vi "FGV_UserMenu.vi"(7 "Command":enum16{"Initialize", "Set", "Get"}(ring), 10 "Use Info":string, 11 "VI Refnum":refnum<vi>) -> (2 "String":string)   [LabVIEW 2017]
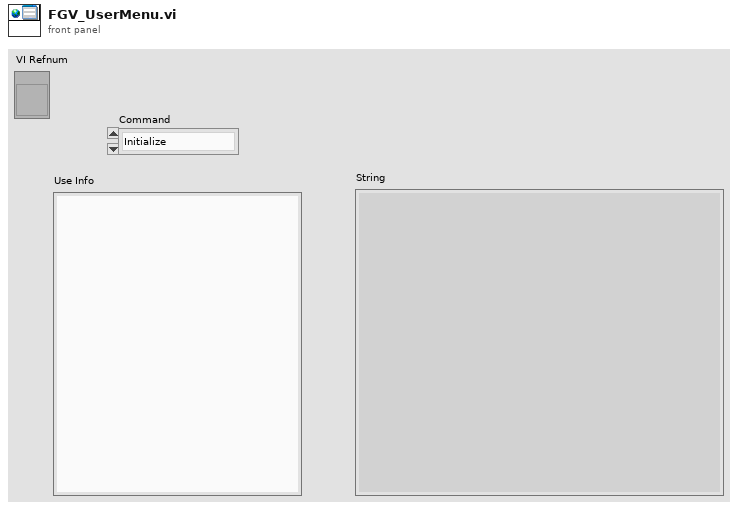
[diagram p1: front panel]
types:
  T1 = cluster{"VI Refnum":refnum<vi>, "Use Info":string}[]
  T2 = cluster{"VI Refnum":refnum<vi>, "Use Info":string}
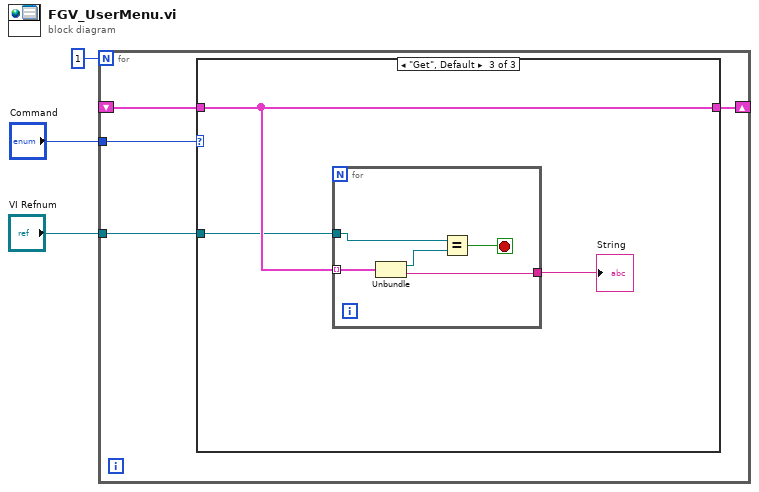
[diagram p0: block diagram]
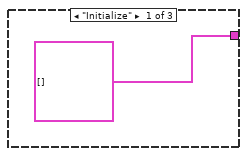
[diagram p2: hidden frame]
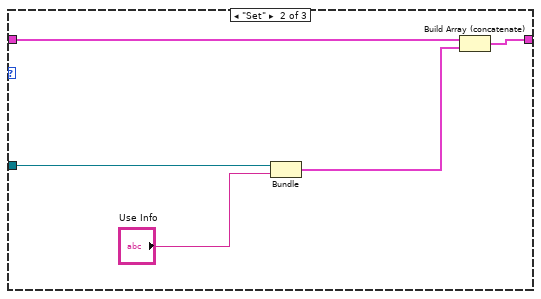
[diagram p3: hidden frame]
diagram:
  n1 = for {
    N: 1 -> [_]
    shift-right: [w4] -> _
    shift-left: _ -> [w7]
    tunnel: "Command" -> [w6]
    tunnel: "VI Refnum" -> [w5]
    n2 = case shown="\"Get\", Default" w6 {
      tunnel: w7 -> [_ w9 w16]
      tunnel: w5 -> [_ w13 w15]
      tunnel: [T1 [] w10 w16] -> w4
      frame "Initialize" {
      }
      frame "Set" {
        n3 = Bundle("VI Refnum"=w13, "Use Info"="Use Info") -> (w11:T2)  [unwired: 1 in]
        n4 = Build Array (concatenate)(w9, w11) -> (w10:T1)
      }
      frame "Get", Default {
        n5 = for {
          tunnel: w16 -> [w21] mode=indexing
          tunnel: w15 -> [w20]
          tunnel: [w17] -> w14
          stop <- w18 stop-if-true
          n6 = Unbundle(w21) -> ("VI Refnum"=w19:refnum<vi>, "Use Info"=w17:string)
          n7 = Equal?(x=w20, y=w19) -> (x = y?=w18:bool)
        }
        "String" <- w14
      }
    }
  }
